vi "cmwtestLV14.vi"() -> ()   [LabVIEW 2014]
uses:
  <userlib>/_RADE/RIO/CMW/classes/CMWGet/openCMWGet.vi
  <userlib>/_RADE/RIO/CMW/classes/CMWGet/CMWGet.vi
  <userlib>/_RADE/RIO/CMW/classes/CMWGet/CMWGet.lvclass
panel:
  out "value":sgl
  out "error out":errorcluster
  in  "error in (no error)":errorcluster
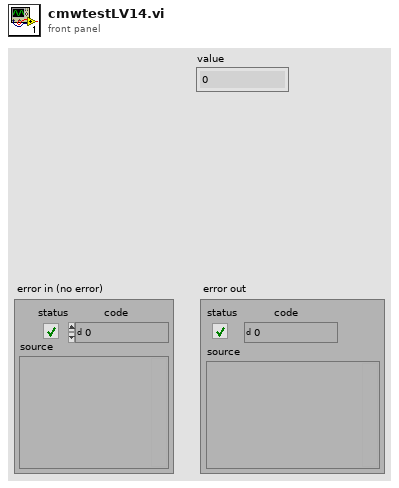
[diagram p1: front panel]
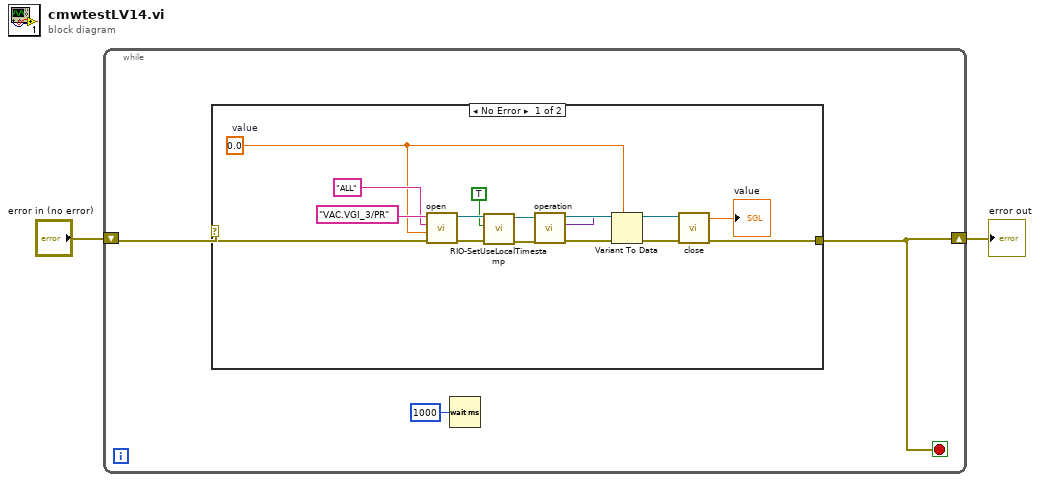
[diagram p0: block diagram]
diagram:
  n1 = while {
    shift-right: [w3] -> w2
    shift-left: "error in (no error)" -> [w5]
    stop <- w3 stop-if-true
    n2 = case shown="No Error" w5 {
      selector: w5 -> [w16 w21]
      tunnel: [w15 w21] -> w3
      frame No Error {
        w6 = sgl 0.0  # value
        n3 = call-poly <userlib>:"open.vi"("error in (no error)"=w16, "Data type"=w6, "Cycle"="ALL", "URL"="VAC.VGI_3/PR") -> ("error out"=w11:errorcluster, "Object out"=w8:refnum<class "CMWGet.lvclass">)  [unwired: 6 in]
        n4 = call-dynamic "RIO-SetUseLocalTimestamp.vi"("error in (no error)"=w11, "Use Local Timestamp?"=TRUE, "CMWBase in"=w8) -> ("error out"=w10:errorcluster, "CMWBase out"=w9:refnum<class "CMWGet.lvclass">)  [unwired: 7 in]
        n5 = call-poly <userlib>:"operation.vi"("error in (no error)"=w10, "Object in"=w9) -> ("error out"=w14:errorcluster, "Data out"=w17:variant, "Object out"=w20:refnum<class "CMWGet.lvclass">)  [unwired: 6 in, 1 out]
        n6 = Variant To Data(error in=w14, type=w6, Variant=w17) -> (data=→"value":sgl, error out=w13:errorcluster)
        n7 = call-dynamic "close.vi"("error in (no error)"=w13, "Object in"=w20) -> ("error out"=w15:errorcluster)  [unwired: 9 in]
      }
      frame Error {
      }
    }
    n8 = Wait (ms)(milliseconds to wait=u32 1000) -> ()  [unwired: 1 out]
  }
  "error out" <- w2
